vi "get update log.vi"(8 "error in (no error)":errorcluster caption="错误输入（无错误）", 11 "服务器信息":T1={"host"="27.154.58.30", "port"=8020, "user"="std", "password"="std23506", "远端地址"="/微站/室外总磷总氮高压过滤无主板新电路板/一体化微型水质监测站.exe"}) -> (0 "error out":errorcluster caption="错误输出", 1 "部分更新日志":string, 2 "remote File Version":string, 3 "更新日志":string)   [LabVIEW 2016, in "update.lvlib"]
uses:
  update.lvlib
  <vilib>/regexp/Match Regular Expression.xnode
  <vilib>/httpClient/LabVIEWHTTPClient.lvlib
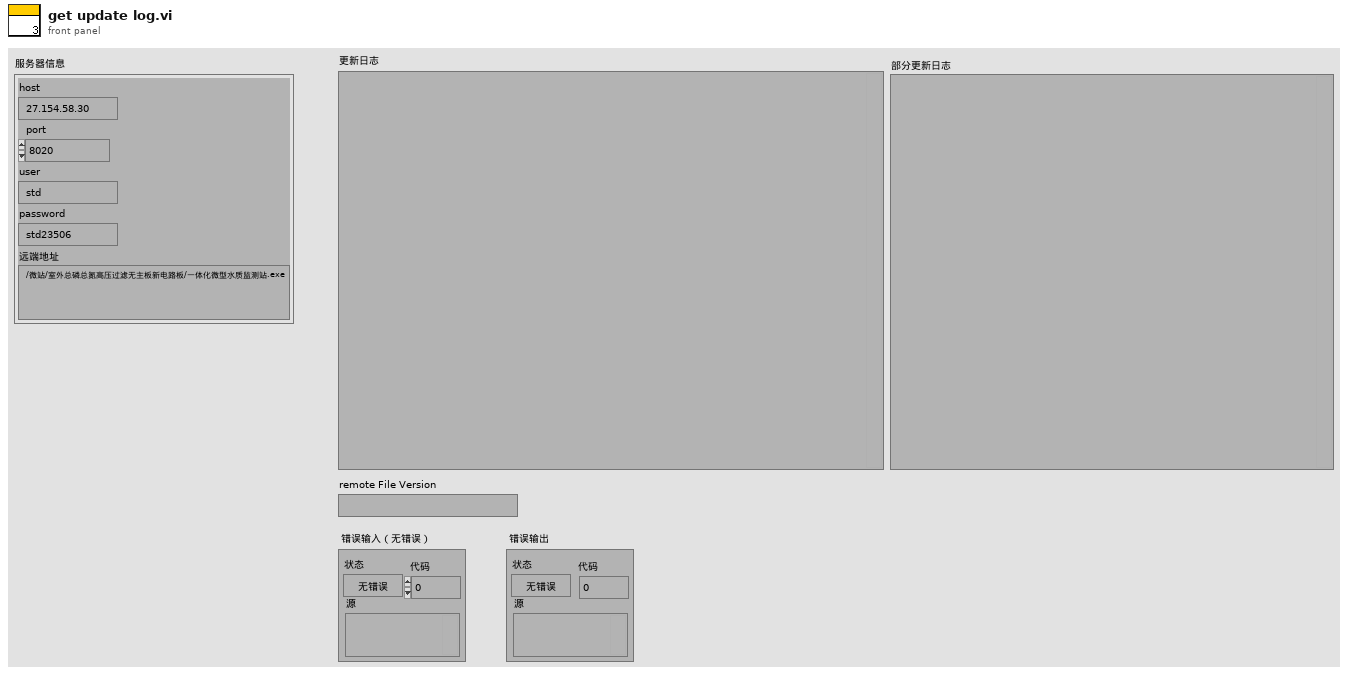
[diagram p1: front panel]
types:
  T1 = cluster{"host":string, "port":u16, "user":string, "password":string, "远端地址":string}
  T2 = typedef "LabVIEWHTTPClient.lvlib/ClientHandle.ctl" = refnum<k1>
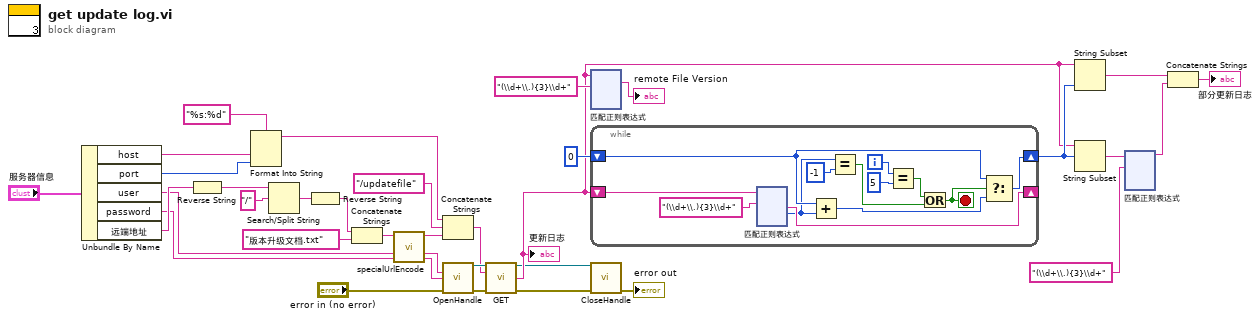
[diagram p0: block diagram]
diagram:
  n1 = Unbundle By Name("服务器信息") -> ("host"=w9:string, "port"=w8:u16, "user"=w12:string, "password"=w13:string, "远端地址"=w19:string)
  n2 = Reverse String(1:w19) -> (0:w30:string)
  n3 = Format Into String(format string="%s:%d" ("格式字符串"), w9, w8) -> (resulting string=w7:string)  [unwired: 2 in, 1 out]
  n4 = Search/Split String(string=w30, search string/char (-)="/" ("搜索字符串/字符(-)")) -> (match + rest of string=w28:string)  [unwired: 1 in, 2 out]
  n5 = Reverse String(1:w28) -> (0:w27:string)
  n6 = Concatenate Strings(w27, "版本升级文档.txt" ("字符串")) -> (w11:string)
  n7 = call "specialUrlEncode.vi"("str"=w11) -> ("UrlEncode"=w10:string)  [unwired: 10 in]
  n8 = Concatenate Strings(w7, "/updatefile", w10) -> (w5:string)
  n9 = call <vilib>:"OpenHandle.vi"("username"=w12, "password"=w13, "error in (no error)"="error in (no error)") -> ("client handle out"=w18:T2, "error out"=w17:errorcluster)  [unwired: 11 in]
  n10 = call <vilib>:"GET.vi"("client handle"=w18, "url"=w5, "error in (no error)"=w17) -> ("client handle out"=w1:T2, "body"=w16:string, "error out"=w3:errorcluster)  [unwired: 9 in, 1 out]
  "更新日志" <- w16
  n11 = xnode "匹配正则表达式"("输入字符串"=w16, "正则表达式"="(\\d+\\.){3}\\d+") -> ("所有匹配"=→"remote File Version":string)  [unwired: 4 in, 4 out]
  n12 = while {
    shift-right: [w43] -> _
    shift-left: w16 -> [w45]
    shift-right: [w44] -> w23
    shift-left: 0 ("匹配后偏移量") -> [w41]
    i -> [w40]
    stop <- w39 stop-if-true
    n13 = xnode "匹配正则表达式"("输入字符串"=w45, "正则表达式"="(\\d+\\.){3}\\d+") -> ("匹配之后"=w43:string, "匹配后偏移量"=w34:i32)  [unwired: 4 in, 3 out]
    n14 = Add(x=w41, y=w34) -> (x+y=w42:i32)
    n15 = Equal?(x=w34, y=-1) -> (x = y?=w36:bool)
    n16 = Equal?(x=w40, y=5) -> (x = y?=w38:bool)
    n17 = Or(x=w38, y=w36) -> (x .or. y?=w39:bool)
    n18 = Select(t=w41, s=w39, f=w42) -> (s? t:f=w44:i32)
  }
  n19 = call <vilib>:"CloseHandle.vi"("client handle"=w1, "error in (no error)"=w3) -> ("error out"=→"error out":errorcluster)  [unwired: 13 in]
  n20 = String Subset(string=w16, length (rest)=w23) -> (substring=w21:string)  [unwired: 1 in]
  n21 = String Subset(string=w16, offset (0)=w23) -> (substring=w24:string)  [unwired: 1 in]
  n22 = xnode "匹配正则表达式"("输入字符串"=w24, "正则表达式"="(\\d+\\.){3}\\d+") -> ("匹配之前"=w22:string)  [unwired: 4 in, 4 out]
  n23 = Concatenate Strings(w21, w22) -> (→"部分更新日志":string)
